vi "PH_Beamline.Calc PA State.vi"(0 "i ref in":refnum<vi>, 5 "error in (no error)":errorcluster) -> (14 "i ref out":refnum<vi>, 17 "PA Exit closed or shining into LL":bool, 18 "PA Exit closed":bool, 19 "error out":errorcluster)   [LabVIEW 2014, in "PH_Beamline.lvlib"]
doc: "THIS VI calculates the PreAmp state of the Beamline"
uses:
  PH_Beamline.lvlib
  PH_Beamline.6P 4 Pos Selector Instances.ctl
  PH_4_Pos_Selector/PH_4_Pos_Selector.Position Selector.ctl
  PH_Common/PH_Common.lvlib
  PH_SystemInformation/PH_SystemInformation.lvlib
  PH_BL-Master/PH_BL-Master.lvlib
  PH_4_Pos_Selector/PH_4_Pos_Selector.lvlib
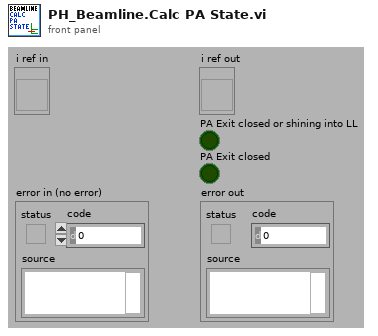
[diagram p1: front panel]
types:
  T1 = enum16{"Laser", "PreAmp", "MainAmp", "Exp 1", "Exp 2", "Exp 3", "Exp 4"}
  T2 = typedef "PH_Beamline.lvlib/PH_Beamline.i attribute.ctl" = cluster{"GUI Refs":cluster{"PA ok":refnum<vi>, "MA ok":refnum<vi>, "fs FE ok":refnum<vi>, "ns FE ok":refnum<vi>, "PA ED ok":refnum<vi>, "MAS ok":refnum<vi>, "Booster ok":refnum<vi>, "Mirrortower ok":refnum<vi>, "In.-Box ok":refnum<vi>, "Compressor ok":refnum<vi>, "Experiment LB ok":refnum<vi>, "Experiment LL ok":refnum<vi>, "PHELIX_Beckhoff_Watchdog":refnum<vi>, "Shutters closed":refnum<vi>, "uOPA ok":refnum<vi>, "Vacuum no shotcond Comp LB":refnum<vi>}, "Refs BL MA":refnum<vi>[], "Refs BL MA-IB":refnum<vi>[], "Refs BL fs":refnum<vi>[], "Refs BL PA ED":refnum<vi>[], "Refs BL MAS":refnum<vi>[], "Refs BL Boo":refnum<vi>[], "Refs BL ns":refnum<vi>[], "Refs BL Mirrortower":refnum<vi>[], "Refs BL Compressor":refnum<vi>[], "Refs BL Exp LB":refnum<vi>[], "Radiation Safety":cluster{"Exp Laserbay":cluster{"Ref Op Mode":refnum<vi>, "Ref Laserbay evacuated":refnum<vi>, "Tagname LB evacuated":string, "Shot Mode":T3, "Laserbay evacuated?":i32, "Tagname HV room locked":string, "HV room locked?":i32, "Ref HV room locked":refnum<vi>, "Tagname bridged?":string, "Ref Bridge":refnum<vi>, "I<1E18W/cm²":bool}, "Exp Laserlab":cluster{"Ref Op Mode":refnum<vi>, "Ref Laserlab evacuated":refnum<vi>, "Tagname LL evacuated":string, "Shot Mode":T3, "Laserlab evacuated?":i32, "Tagname bridged?":string, "Ref Bridge":refnum<vi>, "I<1E18W/cm²":bool}}, "Refs BL LL":refnum<vi>[], "PP Igni Heating GUI Refs":refnum<vi>[], "PP Igni Heating Tagnames ":string[], "Refs BL PA":cluster{"undelayed Line before Shutter":refnum<vi>[], "undelayed Line after Shutter":refnum<vi>[], "before Bypass":refnum<vi>[], "delayed Line before Shutter":refnum<vi>[], "delayed Line after Shutter":refnum<vi>[], "before Shutter Input":refnum<vi>[], "after Shutter Input":refnum<vi>[], "Bypass":refnum<vi>[], "before Shutter Exit":refnum<vi>[], "after Shutter Exit":refnum<vi>[], "to MA":refnum<vi>[], "to Lab":refnum<vi>[]}, "BL":cluster{"YLF_BL_Status":i32, "fs_BL_Status":i32, "fs_YLF_BL_Status":i32, "ns_BL_Status":i32, "PA_Input_BL_Status":i32, "PA_UnDelay_BL_Status":i32, "PA_Delay_BL_Status":i32, "PA_BL_Status":i32, "PA_Bypass_BL_Status":i32, "PA_Exit_BL_Status":i32, "PA_LL_BL_Status":i32, "LL_BL_Status":i32, "PA_MA_BL_Status":i32, "MA_Exit_BL_Status":i32, "MA_Z6_BL_Status":i32, "Z6_BL_Status":i32, "MA_LB_BL_Status":i32, "LB_TB2_BL_Status":i32, "PA_before_Bypass_BL_Status":i32, "LB_TB3_BL_Status":i32}, "State Subsystems":cluster{"PA":bool, "MA":bool, "ns FE":bool, "fs FE":bool, "PA ED":bool, "In.-Box":bool, "MAS":bool, "Booster":bool, "Mirrortower":bool, "Compressor":bool, "Experiment LB":bool, "Experiment LL":bool, "uOPA":bool}, "Status Subscriber Information":T4, "Refs BL uOPA":refnum<vi>[], "PA_Input_2_Beam_6PWpGUI not linked?":bool, "PA_Input_Delay_6PGUI not linked?":bool, "Settings":T7}
  T3 = typedef "PH_Beamline.lvlib/PH_Beamline.Operation Mode.ctl" = i32
  T4 = typedef "PH_Beamline.lvlib/PH_Beamline.Status Subscriber Information.ctl" = cluster{"fs Swich YLF":T5, "fs Exit Shutter":T5, "ns Exit Shutter":T5, "PA Input Shutter":T5, "PA PC WP":T5, "PA PC WP 2":T5, "PA Bypass In":T5, "PA Bypass Out":T5, "PA CH 1":T5, "PA delayed":T5, "PA non delayed":T5, "PA Exit Shutter":T5, "PA Switch Lab":T5, "PA Bridge CH Input MA":T5, "MA Diffusor IB":T5, "MA IB Ready":T5, "MA CH 1":T5, "MA CH 2":T5, "MA CH 3":T5, "MA CH 4":T5, "MA Shutter Align Cam":T5, "MA Position MM5":T5, "Calorimeter Switch":T5, "BL Z6 CH 9":T5, "BL Z6 Beamdump":T5, "BL Z6 Shutter":T5, "COS Sensitivity Switch":T5, "Exp LB Shutter":T5, "Exp LB TB 2":T5, "Exp LB TB 3":T5, "PA LL Input CH":T5, "PA LL Output CH":T5, "LL Comp Input Shutter":T5, "LL Comp Output Shutter":T5, "LL Comp FF Shutter":T5, "Exp LL Shutter":T5, "MA IM In IB":T5, "MA IM Out IB":T5, "MA DB In IB":T5, "MA DB Out IB":T5, "Exp LB Shutter Interlock":T5, "Exp LL Shutter Interlock":T5, "MM1 Force Sensor":T5}
  T5 = typedef "PH_BL-Master.lvlib/PH_BL-Master.Status Subscriber Information.ctl" = cluster{"Index of element":i32, "Attributeset":T6}
  T6 = typedef "PH_BL-Master.lvlib/PH_BL-Master.Attribute Set.ctl" = enum16{"Boolean Status Service Subscriber", "Picture Status Service Subscriber"}
  T7 = typedef "PH_Beamline_Chief.lvlib/PH_Beamline_Chief.Settings.ctl" = cluster{"PA Doublepass Mode":bool, "Compressor Vaccuum LB not relevant":bool, "Windowshutter TB2 not relevant":bool, "Windowshutter TB3 not relevant":bool}
  T8 = typedef "PH_SystemInformation.lvlib/PH_SystemInformationEnabling State.ctl" = i32
  T9 = typedef "PH_Beamline.lvlib/PH_Beamline.6P 4 Pos Selector Instances.ctl" = string
  T10 = enum16{"All, Default", "PreAmp", "MainAmp", "Compressor", "Experiment", "Z6 Telescope"}
  T11 = typedef "PH_4_Pos_Selector.lvlib/PH_4_Pos_Selector.Position Selector.ctl" = u16
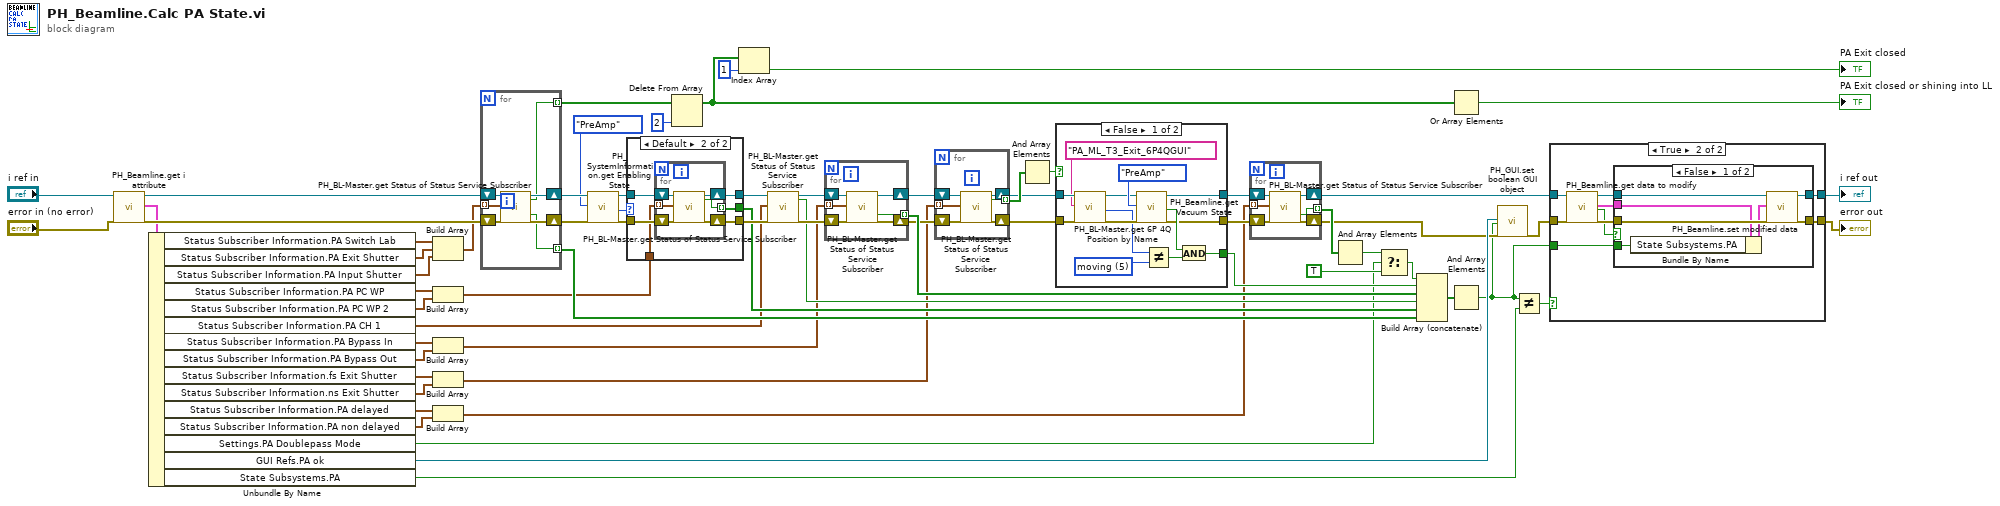
[diagram p0: block diagram]
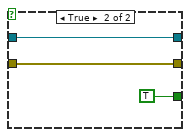
[diagram p2: hidden frame]
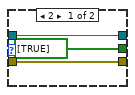
[diagram p3: hidden frame]
diagram:
  n1 = call "PH_Beamline.get i attribute.vi"("i ref in"="i ref in", "error in (no error)"="error in (no error)") -> ("i ref out"=w33:refnum<vi>, "i attribute"=w28:T2, "error out"=w31:errorcluster)  [unwired: 15 in]
  n2 = Unbundle By Name(w28) -> ("Status Subscriber Information.PA Switch Lab"=w14:T5, "Status Subscriber Information.PA Exit Shutter"=w13:T5, "Status Subscriber Information.PA Input Shutter"=w12:T5, "Status Subscriber Information.PA PC WP"=w17:T5, "Status Subscriber Information.PA PC WP 2"=w16:T5, "Status Subscriber Information.PA CH 1"=w18:T5, "Status Subscriber Information.PA Bypass In"=w21:T5, "Status Subscriber Information.PA Bypass Out"=w20:T5, "Status Subscriber Information.fs Exit Shutter"=w24:T5, "Status Subscriber Information.ns Exit Shutter"=w23:T5, "Status Subscriber Information.PA delayed"=w27:T5, "Status Subscriber Information.PA non delayed"=w26:T5, "Settings.PA Doublepass Mode"=w5:bool, "GUI Refs.PA ok"=w29:refnum<vi>, "State Subsystems.PA"=w30:bool)
  n3 = Build Array(w14, w13, w12) -> (w11:T5[])
  n4 = Build Array(w17, w16) -> (w15:T5[])
  n5 = Build Array(w21, w20) -> (w19:T5[])
  n6 = Build Array(w24, w23) -> (w22:T5[])
  n7 = Build Array(w27, w26) -> (w25:T5[])
  n8 = for {
    tunnel: w11 -> [w69] mode=indexing
    shift-right: [w73] -> w53
    shift-left: w31 -> [w70]
    shift-right: [w72] -> w44
    shift-left: w33 -> [w71]
    tunnel: [w68] -> w60 mode=indexing
    tunnel: [w67] -> w10 mode=indexing
    n9 = call "PH_BL-Master.get Status of Status Service Subscriber.vi"("i ref in"=w71, "Wanted Status Subscriber Information"=w69, "error in (no error)"=w70) -> ("i ref out"=w72:refnum<vi>, "off/false/out?"=w67:bool, "off/false/out or on/true/in?"=w68:bool, "error out"=w73:errorcluster)  [unwired: 11 in, 2 out]
  }
  n10 = call "PH_SystemInformation.get Enabling State.vi"("i ref in"=w44, "Wanted State"=T1."PreAmp", "error in (no error)"=w53) -> ("i ref out"=w43:refnum<vi>, "Enabling State"=w41:T8, "error out"=w45:errorcluster)  [unwired: 14 in]
  n11 = case shown="Default" w41 {
    tunnel: [w75 w82] -> w52
    tunnel: [w76 w81] -> w51
    tunnel: [bool[] [TRUE] w80] -> w50
    tunnel: w45 -> [w75 w79]
    tunnel: w43 -> [w76 w78]
    tunnel: w15 -> [_ w77]
    frame 2 {
    }
    frame Default {
      n12 = for {
        tunnel: w77 -> [w84] mode=indexing
        shift-right: [w88] -> w82
        shift-left: w79 -> [w85]
        shift-right: [w87] -> w81
        shift-left: w78 -> [w86]
        tunnel: [w83] -> w80 mode=indexing
        n13 = call "PH_BL-Master.get Status of Status Service Subscriber.vi"("i ref in"=w86, "Wanted Status Subscriber Information"=w84, "error in (no error)"=w85) -> ("i ref out"=w87:refnum<vi>, "off/false/out?"=w83:bool, "error out"=w88:errorcluster)  [unwired: 11 in, 3 out]
      }
    }
  }
  n14 = Delete From Array(array=w10, index=2) -> (array with subset deleted=w8:bool[])  [unwired: 1 in, 1 out]
  n15 = Index Array(array=w8, index=1) -> (element=→"PA Exit closed":bool)
  n16 = call "PH_BL-Master.get Status of Status Service Subscriber.vi"("i ref in"=w51, "Wanted Status Subscriber Information"=w18, "error in (no error)"=w52) -> ("i ref out"=w62:refnum<vi>, "off/false/out?"=w61:bool, "error out"=w63:errorcluster)  [unwired: 11 in, 3 out]
  n17 = for {
    tunnel: w19 -> [w90] mode=indexing
    shift-right: [w93] -> w36
    shift-left: w63 -> [w94]
    shift-right: [w91] -> w38
    shift-left: w62 -> [w92]
    tunnel: [w89] -> w64 mode=indexing
    n18 = call "PH_BL-Master.get Status of Status Service Subscriber.vi"("i ref in"=w92, "Wanted Status Subscriber Information"=w90, "error in (no error)"=w94) -> ("i ref out"=w91:refnum<vi>, "off/false/out or on/true/in?"=w89:bool, "error out"=w93:errorcluster)  [unwired: 11 in, 3 out]
  }
  n19 = for {
    shift-right: [w95] -> w37
    shift-left: w38 -> [w100]
    shift-right: [w96] -> w35
    shift-left: w36 -> [w99]
    tunnel: w22 -> [w98] mode=indexing
    tunnel: [w97] -> w40 mode=indexing
    n20 = call "PH_BL-Master.get Status of Status Service Subscriber.vi"("i ref in"=w100, "Wanted Status Subscriber Information"=w98, "error in (no error)"=w99) -> ("i ref out"=w95:refnum<vi>, "off/false/out?"=w97:bool, "error out"=w96:errorcluster)  [unwired: 11 in, 3 out]
  }
  n21 = And Array Elements(Boolean array=w40) -> (logical AND=w39:bool)
  n22 = case shown="False" w39 {
    tunnel: [w103 TRUE ("vacua in range")] -> w65
    tunnel: w37 -> [w109 w116]
    tunnel: w35 -> [w107 w115]
    tunnel: [w111 w115] -> w59
    tunnel: [w110 w116] -> w58
    frame False {
      w104 = T11 5 items=["unknown", "Position I", "Position II", "Position III", "Position IV", "moving"] ("y")
      n23 = call "PH_BL-Master.get 6P 4Q Position by Name.vi"("i ref in"=w109, "6P 4Q Instance"=T9 "PA_ML_T3_Exit_6P4QGUI" ("6P 4 Pos Selector Instances"), "error in (no error)"=w107) -> ("i ref out"=w108:refnum<vi>, "Position"=w105:T11, "error out"=w106:errorcluster)  [unwired: 10 in, 4 out]
      n24 = call "PH_Beamline.get Vacuum State.vi"("i ref in"=w108, "Subsystem"=T10."PreAmp", "error in (no error)"=w106) -> ("i ref out"=w110:refnum<vi>, "vacua in range"=w112:bool, "error out"=w111:errorcluster)  [unwired: 14 in]
      n25 = Not Equal?(x=w105, y=w104) -> (x != y?=w102:bool)
      n26 = And(x=w112, y=w102) -> (x .and. y?=w103:bool)
    }
    frame True {
    }
  }
  n27 = for {
    tunnel: w25 -> [w118] mode=indexing
    shift-right: [w122] -> w3
    shift-left: w59 -> [w119]
    shift-right: [w121] -> w4
    shift-left: w58 -> [w120]
    tunnel: [w117] -> w57 mode=indexing
    n28 = call "PH_BL-Master.get Status of Status Service Subscriber.vi"("i ref in"=w120, "Wanted Status Subscriber Information"=w118, "error in (no error)"=w119) -> ("i ref out"=w121:refnum<vi>, "off/false/out or on/true/in?"=w117:bool, "error out"=w122:errorcluster)  [unwired: 11 in, 3 out]
  }
  n29 = And Array Elements(Boolean array=w57) -> (logical AND=w56:bool)
  n30 = Select(t=w56, s=w5, f=TRUE) -> (s? t:f=w55:bool)
  n31 = Build Array (concatenate)(w55, w65, w64, w61, w50, w60) -> (w66:bool[])
  n32 = Or Array Elements(Boolean array=w8) -> (logical OR=→"PA Exit closed or shining into LL":bool)
  n33 = And Array Elements(Boolean array=w66) -> (logical AND=w2:bool)
  n34 = call "PH_GUI.set boolean GUI object.vi"("Boolean Knob GUI Ref"=w29, "Value"=w2, "error in (no error)"=w3) -> ("error out"=w47:errorcluster)  [unwired: 16 in]
  n35 = Not Equal?(x=w2, y=w30) -> (x != y?=w49:bool)
  n36 = case shown="True" w49 {
    tunnel: w4 -> [w124 w129]
    tunnel: [w124 w128] -> w48
    tunnel: w47 -> [w123 w127]
    tunnel: [w123 w126] -> w46
    tunnel: w2 -> [_ w125]
    frame False {
    }
    frame True {
      n37 = call "PH_Beamline.get data to modify.vi"("i ref in"=w129, "error in (no error)"=w127) -> ("i ref out"=w132:refnum<vi>, "i attribute"=w130:T2, "timed out"=w131:bool, "error out"=w133:errorcluster)  [unwired: 14 in]
      n38 = case shown="False" w131 {
        tunnel: w133 -> [w140 w141]
        tunnel: w132 -> [w139 w142]
        tunnel: [w138 w141] -> w126
        tunnel: [w137 w142] -> w128
        tunnel: w130 -> [w136 _]
        tunnel: w125 -> [w134 _]
        frame False {
          n39 = Bundle By Name(cluster=w136, "State Subsystems.PA"=w134) -> (w135:T2)
          n40 = call "PH_Beamline.set modified data.vi"("i ref in"=w139, "i attribute"=w135, "error in (no error)"=w140) -> ("i ref out"=w137:refnum<vi>, "error out"=w138:errorcluster)  [unwired: 15 in]
        }
        frame True {
        }
      }
    }
  }
  "i ref out" <- w48
  "error out" <- w46
